vi "Get VIPM Dependency Maps.vi"(7 "Force Reload?(F)":bool, 8 "error in":errorcluster) -> (0 "error out":errorcluster, 1 "Unmatched Packages":string[](array[string]), 2 "External Target Map":map{string, string}(c390), 3 "Internal Target Map":map{string, string}(c390), 5 "Package Array":T1[](array[typedef]))   [LabVIEW 2019, in "Project.Dependencies Finder.lvlib" / "Dependency Source_VIPM.lvclass"]
doc: "Get paths related to all known packages and return them in a map matching them to the package name.\n\n2020-11-11: Henrik Dueholm Hansen"
uses:
  Dependency Source_VIPM.lvclass
  Ctl/Ctl_Package Identifier Cluster.ctl
  ce6ecaaf-38ea-4476-9fc5-063443edb655.vi
  <vilib>/Utility/config.llb/NI_LVConfig.lvlib
panel:
  out "Package Examination Progress":i32(slide) scale=0.0..100.0
  # "New or changed package(s) detected!\nScanning for Path Identifiers. \nThis may take a while."
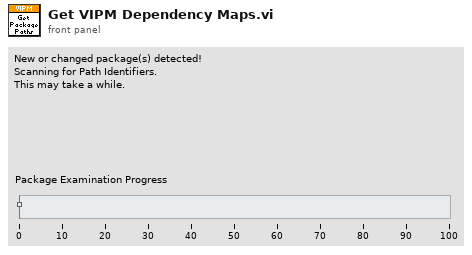
[diagram p1: front panel]
types:
  T1 = typedef "Project.Dependencies Finder.lvlib/Dependency Source_VIPM.lvclass/Ctl_Package Identifier Cluster.ctl" = cluster{"Package Name":string, "Internal Package?":bool, "Newest?":bool, "Version":i32[], "Spec File Name":string, "Spec File MD5":string, "Path Identifiers":string[]}
  T2 = enum32{"Invalid", "Standard", "Closed", "Hidden", "Minimized", "Maximized"}
  T3 = typedef "NI_LVConfig.lvlib/Config Data RefNum.ctl" = refnum<k1>
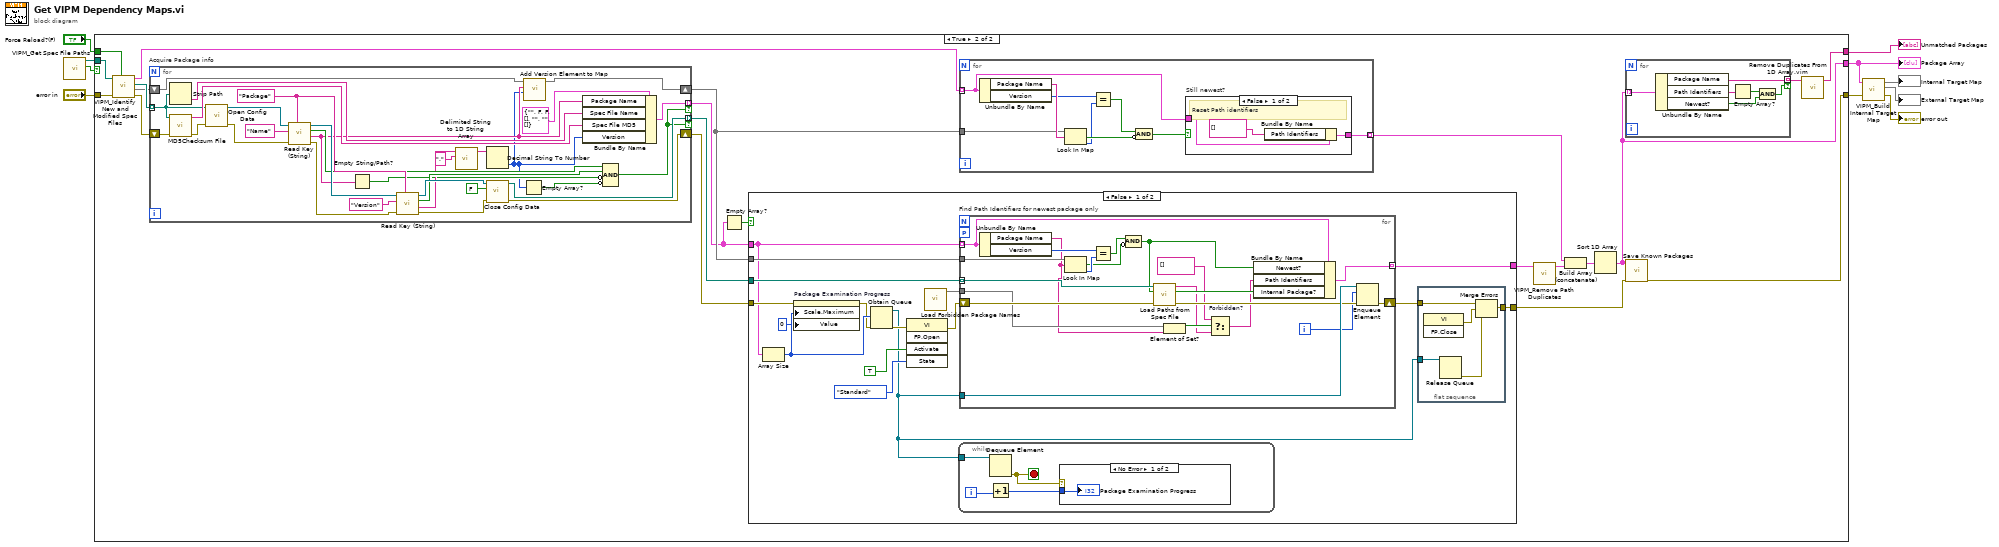
[diagram p0: block diagram]
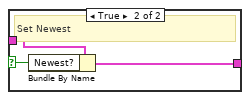
[diagram p5: hidden frame]
diagram:
  n1 = call "VIPM_Get Spec File Paths.vi"() -> ("Success?"=w4:bool, "Spec Paths"=w7:path[])  [unwired: 10 in]
  n2 = case shown="True" w4 {
    tunnel: [w10 w24] -> w8
    tunnel: "error in" -> [w10 w27]
    tunnel: w7 -> [_ w29]
    tunnel: [_ w21] -> w6
    tunnel: [_ w26] -> w5
    tunnel: "Force Reload?(F)" -> [_ w23]
    frame False {
    }
    frame True {
      n3 = call "VIPM_Identify New and Modified Spec Files.vi"("Force Reload?(F)"=w23, "error in (no error)"=w27, "Spec Files"=w29) -> ("error out"=w20:errorcluster, "Version map"=w16:map{string, i32[]}, "New or Modified Spec Files"=w18:path[], "Unchanged Package Array"=w14:T1[])  [unwired: 5 in]
      n4 = for "Acquire Package info" {
        tunnel: w18 -> [w121] mode=indexing
        tunnel: [w104] -> w17 mode=indexing if=w100
        tunnel: [w101] -> w12 mode=indexing if=w100
        shift-right: [w99] -> w19
        shift-left: w20 -> [w119]
        shift-right: [w96] -> w15
        shift-left: w16 -> [w98]
        w112 = "Package"
        n5 = Strip Path(path=w121) -> (name=w124:string)  [unwired: 1 out]
        n6 = call <vilib>:"MD5Checksum File.vi"("error in (no error)"=w119, "Path"=w121) -> ("error out"=w118:errorcluster, "MD5 message-digest"=w123:string)  [unwired: 8 in]
        n7 = call <vilib>:"Open Config Data.vi"("error in (no error)"=w118, "configuration file path"=w121) -> ("error out"=w117:errorcluster, "refnum"=w120:T3)  [unwired: 7 in, 1 out]
        n8 = call <vilib>:"Read Key (String).vi"("section"=w112, "error in (no error)"=w117, "key"="Name", "refnum"=w120) -> ("error out"=w116:errorcluster, "value"=w97:string, "found?"=w110:bool, "refnum out"=w115:T3)  [unwired: 4 in]
        n9 = Empty String/Path?(string/path=w97) -> (empty?=w103:bool)
        n10 = call <vilib>:"Read Key (String).vi"("section"=w112, "error in (no error)"=w116, "key"="Version", "refnum"=w115) -> ("error out"=w105:errorcluster, "value"=w108:string, "found?"=w109:bool, "refnum out"=w114:T3)  [unwired: 4 in]
        n11 = call <vilib>:"Delimited String to 1D String Array.vi"("delimiter"=".", "delimited string"=w108) -> ("string array"=w106:string[])  [unwired: 9 in]
        n12 = Decimal String To Number(string=w106) -> (number=w95:i32[])  [unwired: 2 in, 1 out]
        n13 = call <vilib>:"Close Config Data.vi"("error in (no error)"=w105, "write file if changed (T)"=FALSE, "refnum"=w114) -> ("error out"=w99:errorcluster, "file path"=w104:path)  [unwired: 7 in]
        n14 = Empty Array?(array=w95) -> (empty?=w102:bool)
        n15 = call "Add Version Element to Map.vi"("Version"=w95, "Package Name"=w97, "Version map in"=w98) -> ("Version map out"=w96:map{string, i32[]})  [unwired: 8 in]
        n16 = Bundle By Name(cluster=T1 {"Package Name"="", "Internal Package?"=FALSE, "Newest?"=FALSE, "Version"=[], "Spec File Name"="", "Spec File MD5"="", "Path Identifiers"=[]}, "Package Name"=w97, "Spec File Name"=w124, "Spec File MD5"=w123, "Version"=w95) -> (w101:T1)
        n17 = Compound Arithmetic op=AND(w110, w109, invert w103, invert w102) -> (w100:bool)
      }
      n18 = Empty Array?(array=w12) -> (empty?=w11:bool)
      n19 = case shown="False" w11 {
        tunnel: [w47 _] -> w31
        tunnel: [w34 w79] -> w25
        tunnel: w19 -> [w44 w79]
        tunnel: w17 -> [w46 _]
        tunnel: w15 -> [w45 _]
        tunnel: w12 -> [w43 _]
        frame False {
          n20 = Array Size(array=w43) -> (size(s)=w42:i32)
          n21 = property on="Package Examination Progress" class="Slide (strict)"(error in=w44, "Scale.Maximum"=w42, "Value"=0 ("Package Examination Progress")) -> (error out=w41:errorcluster)  [unwired: 1 in, 1 out]
          n22 = Obtain Queue(element data type=w42, error in (no error)=w41) -> (queue out=w33:refnum<queue>, error out=w37:errorcluster)  [unwired: 3 in, 1 out]
          n23 = invoke class="VI" method="FP.Open"(error in=w37, "Activate"=TRUE, "State"=T2."Standard") -> (error out=w36:errorcluster)  [unwired: 2 in, 4 out]
          n24 = call "Load Forbidden Package Names.vi"() -> ("Forbidden Packages"=w32:set{string})  [unwired: 11 in]
          n25 = while {
            tunnel: w33 -> [w56]
            i -> [w55]
            stop <- w53 stop-if-true
            n26 = Dequeue Element(queue=w56) -> (error out=w53:errorcluster)  [unwired: 2 in, 3 out]
            n27 = Increment(x=w55) -> (x+1=w54:i32)
            n28 = case shown="No Error" w53 {
              tunnel: w54 -> [w57 _]
              frame No Error {
                "Package Examination Progress" <- w57
              }
              frame Error {
              }
            }
          }
          n29 = for "Find Path Identifiers for newest package only" {
            shift-right: [w66] -> w35
            shift-left: w36 -> [w77]
            tunnel: [w78] -> w47 mode=indexing
            tunnel: w46 -> [w76] mode=indexing
            tunnel: w45 -> [w75]
            tunnel: w43 -> [w74] mode=indexing
            workers-P: _ -> [_]
            tunnel: w33 -> [w68]
            tunnel: w32 -> [w63]
            i -> [w65]
            n30 = Unbundle By Name(w74) -> ("Package Name"=w62:string, "Version"=w73:i32[])
            n31 = Look In Map(map=w75, key=w62) -> (key not found?=w70:bool, value=w72:i32[])  [unwired: 1 in]
            n32 = Equal?(x=w73, y=w72) -> (x = y?=w71:bool)
            n33 = Compound Arithmetic op=AND(w71, invert w70) -> (w69:bool)
            n34 = call "Load Paths from Spec File.vi"("error in (no error)"=w77, "Highest Version?"=w69, "Spec path"=w76) -> ("error out"=w67:errorcluster, "Internal Target?"=w64:bool, "External Path Combinations"=w60:string[])  [unwired: 6 in]
            n35 = Element of Set?(10:w62, 11:w63) -> (3:w61:bool)
            n36 = Select "Forbidden?"(t=string[] [], s=w61, f=w60) -> (s? t:f=w58:string[])
            n37 = Bundle By Name(cluster=w74, "Newest?"=w69, "Path Identifiers"=w58, "Internal Package?"=w64) -> (w78:T1)
            n38 = Enqueue Element(queue=w68, element=w65, error in (no error)=w67) -> (error out=w66:errorcluster)  [unwired: 1 in, 2 out]
          }
          n39 = flat-sequence {
            tunnel: w35 -> [w52]
            tunnel: [w51] -> w34
            tunnel: w33 -> [w49]
            frame #0 {
              n40 = invoke class="VI" method="FP.Close"() -> (error out=w50:errorcluster)  [unwired: 3 in, 2 out]
              n41 = Release Queue(queue=w49) -> (error out=w48:errorcluster)  [unwired: 2 in, 2 out]
              n42 = Merge Errors(w52, w50, w48) -> (w51:errorcluster)
            }
          }
        }
        frame True {
        }
      }
      n43 = for {
        tunnel: w14 -> [w80] mode=indexing
        tunnel: w15 -> [w83]
        tunnel: [w81] -> w13 mode=indexing
        n44 = Unbundle By Name(w80) -> ("Package Name"=w88:string, "Version"=w84:i32[])
        n45 = Look In Map(map=w83, key=w88) -> (key not found?=w87:bool, value=w85:i32[])  [unwired: 1 in]
        n46 = Equal?(x=w84, y=w85) -> (x = y?=w86:bool)
        n47 = Compound Arithmetic op=AND(w86, invert w87) -> (w82:bool)
        n48 = case "Still newest?" shown="False" w82 {
          selector: w82 -> [_ w92]
          tunnel: [w89 w93] -> w81
          tunnel: w80 -> [w91 w94]
          frame False {
            # "Reset Path identifiers"
            n49 = Bundle By Name(cluster=w91, "Path Identifiers"=string[] []) -> (w89:T1)
          }
          frame True {
            # "Set Newest"
            n50 = Bundle By Name(cluster=w94, "Newest?"=w92) -> (w93:T1)
          }
        }
      }
      n51 = call "VIPM_Remove Path Duplicates.vi"("Package Array in"=w31) -> ("Package Array out"=w30:T1[])  [unwired: 10 in]
      n52 = Build Array (concatenate)(w13, w30) -> (w28:T1[])
      n53 = Sort 1D Array(array=w28) -> (sorted array=w26:T1[])
      n54 = for {
        tunnel: w26 -> [w131] mode=indexing
        tunnel: [w129] -> w22 mode=indexing if=w127
        n55 = Unbundle By Name(w131) -> ("Package Name"=w129:string, "Path Identifiers"=w130:string[], "Newest?"=w126:bool)
        n56 = Empty Array?(array=w130) -> (empty?=w128:bool)
        n57 = And(x=w128, y=w126) -> (x .and. y?=w127:bool)
      }
      n58 = call "Save Known Packages.vi"("error in (no error)"=w25, "Package Array from File"=w26) -> ("error out"=w24:errorcluster)  [unwired: 8 in, 1 out]
      n59 = call "Remove Duplicates From 1D Array.vim"("array"=w22) -> ("array with duplicates removed"=w21:string[])  [unwired: 10 in]
    }
  }
  "error out" <- w8
  "Unmatched Packages" <- w6
  "Package Array" <- w5
  n60 = call "VIPM_Build Internal Target Map.vi"("Package Array"=w5) -> ("External Target Map"=→"External Target Map":map{string, string}, "Internal Target Map"=→"Internal Target Map":map{string, string})  [unwired: 9 in]
